vi "获取测试数据.vi"(8 "end time":timestamp, 9 "start time":timestamp, 10 "测量模式":string, 11 "table":string) -> (1 "data":T1(array[cluster]), 2 "有数据":bool, 3 "table 2":string)   [LabVIEW 2016, in "环境动力监测库.lvlib" / "NMEA.lvlib"]
uses:
  NMEA.lvlib
  <vilib>/addons/database/_DB Variant To Data/Database Variant To Data.xnode
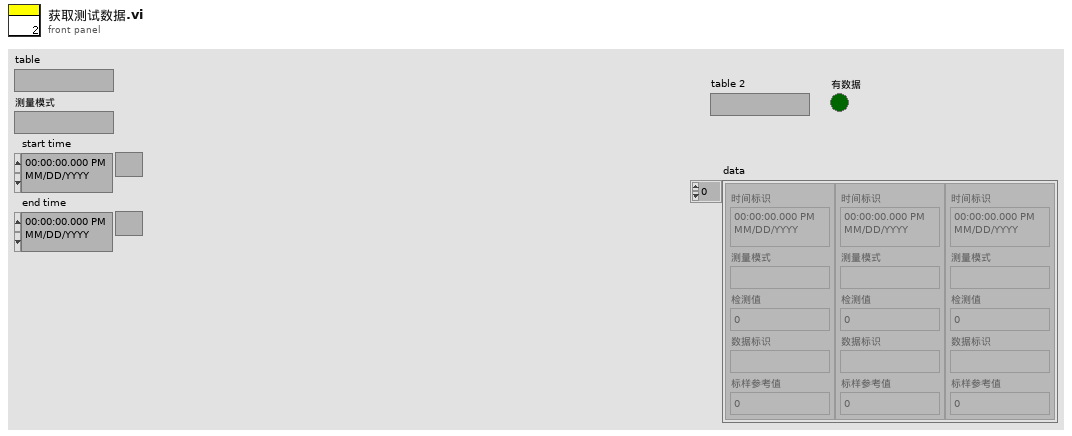
[diagram p1: front panel]
types:
  T1 = cluster{"时间标识":timestamp, "测量模式":string, "检测值":dbl, "数据标识":string, "标样参考值":dbl}[]
  T2 = cluster{"时间标识":timestamp, "测量模式":string, "检测值":dbl, "数据标识":string, "检测值 2":dbl}[]
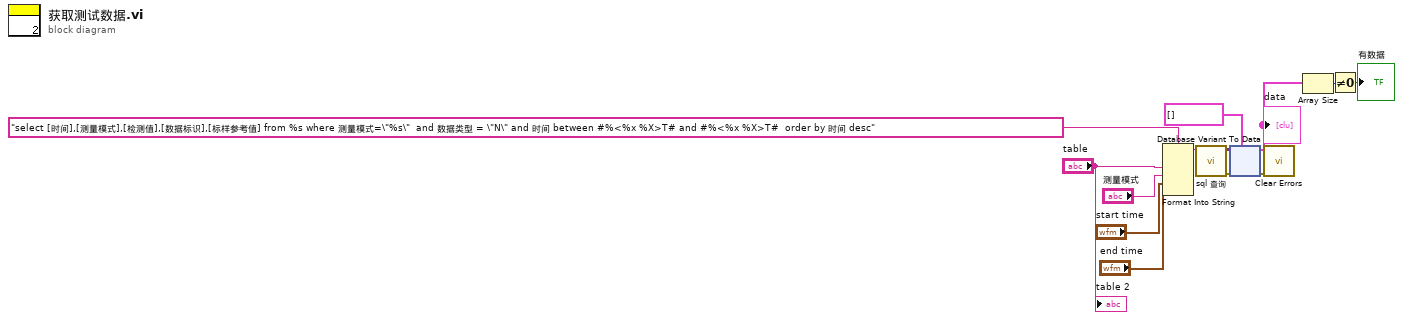
[diagram p0: block diagram]
diagram:
  n1 = Format Into String(format string="select [时间],[测量模式],[检测值],[数据标识],[标样参考值] from %s where 测量模式=\"%s\"  and 数据类型 = \"N\" and 时间 between #%<%x %X>T# and #%<%x %X>T#  order by 时间 desc" ("格式字符串"), "table", "测量模式", "start time", "end time") -> (resulting string=w11:string)  [unwired: 2 in, 1 out]
  n2 = call "sql 查询.vi"("SQL query"=w11) -> ("error out"=w8:errorcluster, "recordset data"=w10:variant[][])  [unwired: 9 in]
  n3 = xnode "Database Variant To Data"("database variant"=w10, "error in (no error)"=w8, "type"=T1 []) -> ("data"=w2:T2, "error out"=w1:errorcluster)
  "data" <- w2
  n4 = call <vilib>:"Clear Errors.vi"("error in (no error)"=w1) -> ()  [unwired: 5 in, 2 out]
  n5 = Array Size(array=w2) -> (size(s)=w4:i32)
  n6 = Not Equal To 0?(x=w4) -> (x != 0?=→"有数据":bool)
  "table 2" <- "table"
